vi "Magna SIC Command Q.vi"(11 "error in (no error)":errorcluster) -> (8 "queue out":refnum<queue>, 15 "error out":errorcluster)   [LabVIEW 2011]
uses:
  Magna Command Definer.ctl
  Magna Commands.ctl
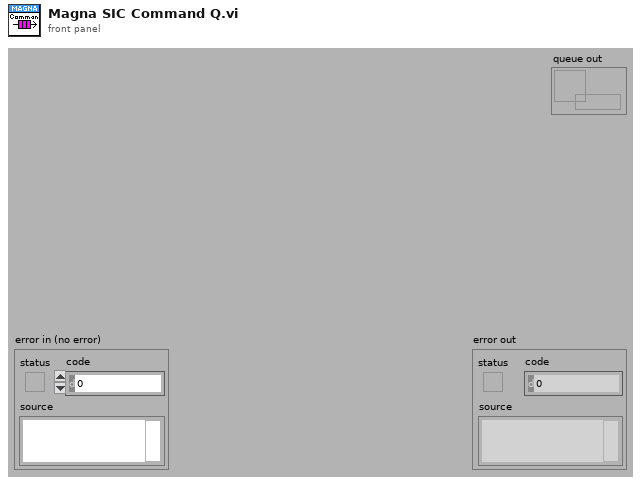
[diagram p1: front panel]
types:
  T1 = typedef "Magna Command Definer.ctl" = cluster{"Action":T2, "n(0)":i32, "d(0.0)":dbl}
  T2 = typedef "Magna Commands.ctl" = enum16{"Read Inputs", "HV ON", "HV OFF", "Set Resistance", "Set Head Voltage SP"}
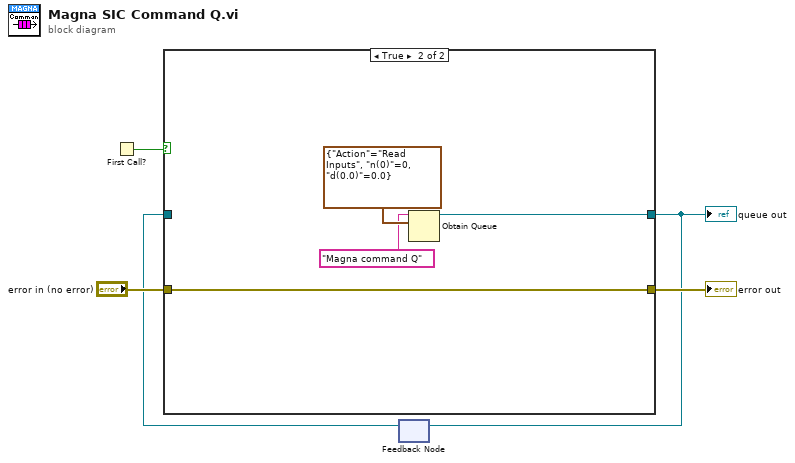
[diagram p0: block diagram]
diagram:
  n1 = First Call?() -> (First Call?: T/F=w3:bool)
  n2 = feedback #1() -> (w1:refnum<queue>)  [unwired: 1 in]
  n3 = case shown="True" w3 {
    tunnel: [w7 w11] -> w5
    tunnel: "error in (no error)" -> [w7 w11]
    tunnel: [w6 w8] -> w2
    tunnel: w1 -> [w6 _]
    frame False {
    }
    frame True {
      n4 = Obtain Queue(name (unnamed)="Magna command Q", element data type=T1 {"Action"=enum."Read Inputs", "n(0)"=0, "d(0.0)"=0.0} ("PCP command")) -> (queue out=w8:refnum<queue>)  [unwired: 3 in, 2 out]
    }
  }
  "error out" <- w5
  "queue out" <- w2
  n5 = feedback-in #1(w2) -> ()
